vi "Delete Data.vi"(8 "error in (no error)":errorcluster, 10 "Rows":i32[](array[numeric]), 11 "MCListbox with Checkboxes in":refnum<class "MCListbox with Checkboxes.lvclass">) -> (0 "error out":errorcluster, 3 "MCListbox with Checkboxes out":refnum<class "MCListbox with Checkboxes.lvclass">)   [LabVIEW 2016, in "MCListbox with Checkboxes.lvclass"]
uses:
  MCListbox with Checkboxes.lvclass
  <userlib>/_OpenG.lib/array/array.llb/Delete Elements from 2D Array (String)__ogtk.vi
  <userlib>/_OpenG.lib/array/array.llb/Delete Elements from 1D Array (Boolean)__ogtk.vi
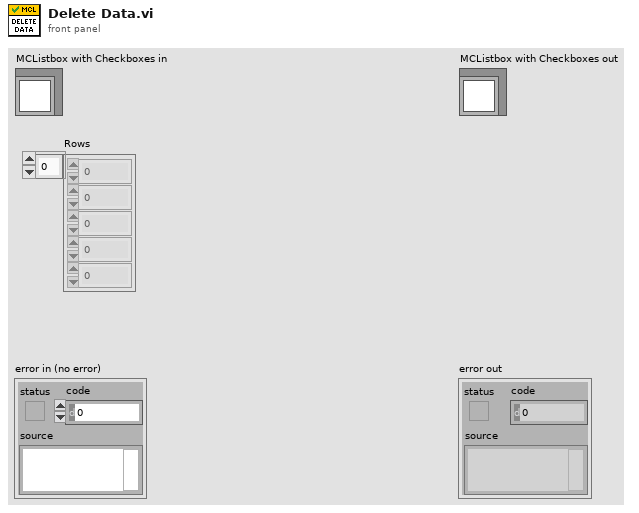
[diagram p1: front panel]
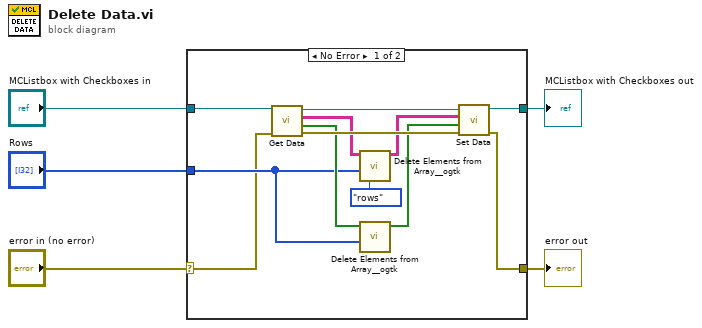
[diagram p0: block diagram]
diagram:
  n1 = case shown="No Error" "error in (no error)" {
    selector: "error in (no error)" -> [w9 w19]
    tunnel: [w13 w19] -> w4
    tunnel: [w14 w18] -> w2
    tunnel: "MCListbox with Checkboxes in" -> [w16 w18]
    tunnel: "Rows" -> [w10 _]
    frame No Error {
      n2 = call "Get Data.vi"("error in (no error)"=w9, "MCListbox with Checkboxes in"=w16) -> ("error out"=w17:errorcluster, "Check Data"=w11:bool[], "Cell Data"=w12:string[][], "MCListbox with Checkboxes out"=w15:refnum<class "MCListbox with Checkboxes.lvclass">)  [unwired: 6 in]
      n3 = call-poly <userlib>:"Delete Elements from Array__ogtk.vi"("delete (rows or columns)"=enum16{"rows", "columns"}."rows", "indices"=w10, "array"=w12) -> ("array w/ subset deleted"=w8:string[][])  [unwired: 7 in, 1 out]
      n4 = call-poly <userlib>:"Delete Elements from Array__ogtk.vi"("indices"=w10, "array"=w11) -> ("array w/ subset deleted"=w7:bool[])  [unwired: 8 in, 1 out]
      n5 = call "Set Data.vi"("error in (no error)"=w17, "Check Data"=w7, "Cell Data"=w8, "MCListbox with Checkboxes in"=w15) -> ("error out"=w13:errorcluster, "MCListbox with Checkboxes out"=w14:refnum<class "MCListbox with Checkboxes.lvclass">)  [unwired: 6 in]
    }
    frame Error {
    }
  }
  "error out" <- w4
  "MCListbox with Checkboxes out" <- w2
